vi "SDCP Receiver and Transmitter - Tx Table Updater.vi"(5 "Current Cell Position":T2, 7 "Entry position descriptors":cluster{"Start Row":i32, "End Row":i32}[](array[cluster]), 8 "error in (no error)":errorcluster, 10 "Table Control":refnum<vi>, 11 "Tx Table entry cluster array in":T1[](array[typedef])) -> (0 "error out":errorcluster, 3 "Tx Table entry cluster array out":T1[](array[typedef]))   [LabVIEW 2020]
uses:
  <vilib>/Utility/miscctls.llb/LVRowAndColumnTypeDef.ctl
  Typedefs/SDCP SMF Receiver and Transmitter - Transmit Table Element.ctl
  Typedefs/SDCP - Standard Message Frame Parameters - FGV - commands.ctl
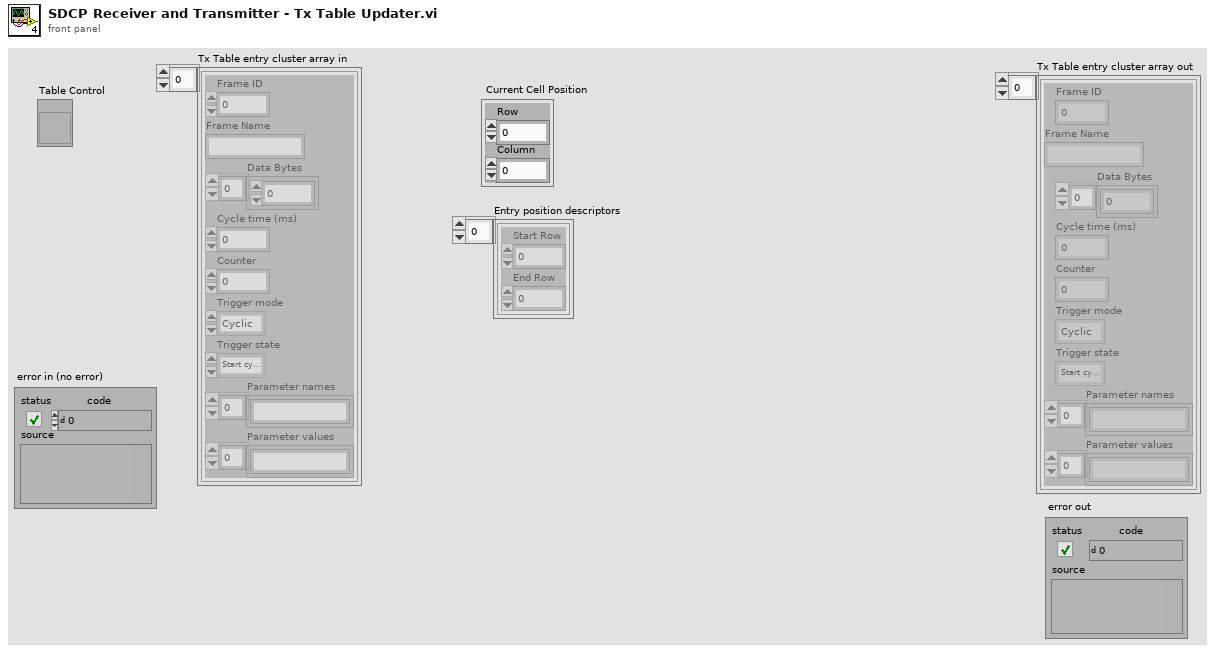
[diagram p1: front panel]
types:
  T1 = typedef "SDCP SMF Receiver and Transmitter - Transmit Table Element.ctl" = cluster{"Frame ID":i32, "Frame Name":string, "Data Bytes":u8[], "Cycle time (ms)":i32, "Counter":i32, "Trigger mode":enum16{"Triggered", "Cyclic"}, "Trigger state":enum16{"Stop cyclic trigger", "Start cyclic trigger", "Stop single trigger", "Start single trigger"}, "Parameter names":string[], "Parameter values":string[]}
  T2 = typedef "LVRowAndColumnTypeDef.ctl" = cluster{"Row":i32, "Column":i32}
  T3 = typedef "SDCP - Standard Message Frame Parameters - FGV - commands.ctl" = enum16{"Write descriptors", "Read descriptors", "Read values", "Load parameters from file", "Write values", "Read all descriptors"}
  T4 = enum16{"Stop cyclic trigger", "Start cyclic trigger", "Stop single trigger", "Start single trigger"}
  T5 = typedef "SDCP - SMF parameter descriptors.ctl" = cluster{"Frame name":string, "Frame ID":i32, "Data type":string, "Start Position":i32, "Length":i32, "Factor":dbl, "Offset":dbl, "Parameter name":string, "Value":string}
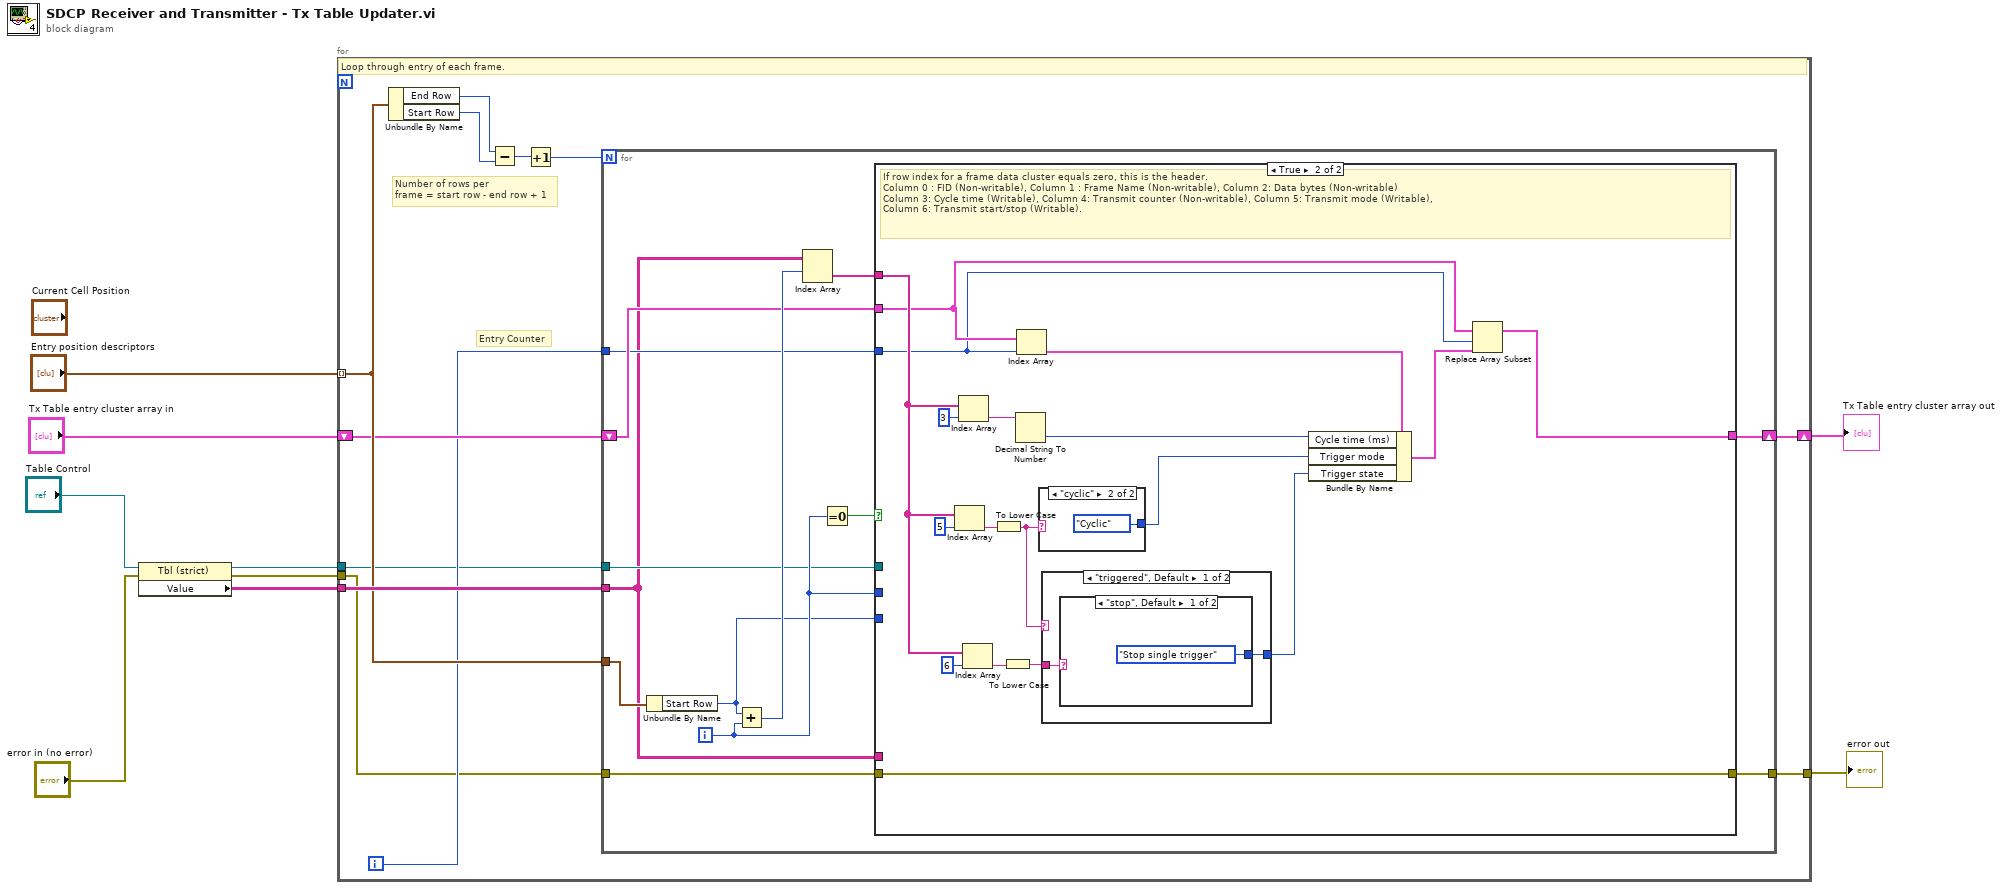
[diagram p0: block diagram]
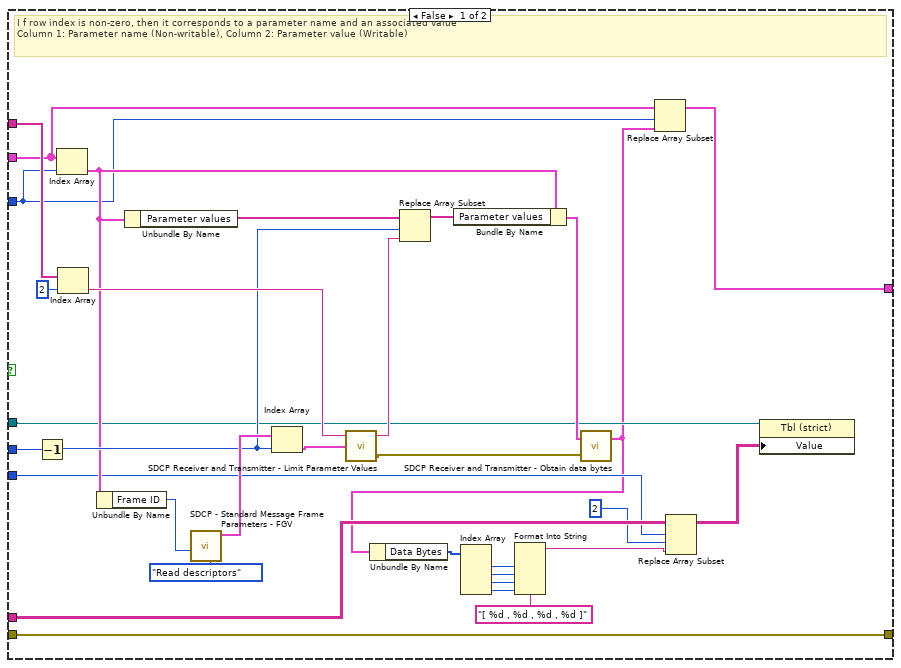
[diagram p2: hidden frame]
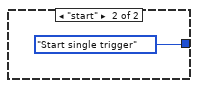
[diagram p3: hidden frame]
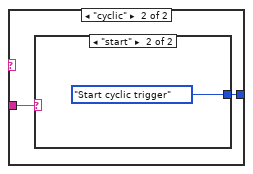
[diagram p4: hidden frame]
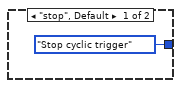
[diagram p5: hidden frame]
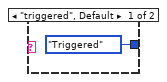
[diagram p6: hidden frame]
diagram:
  n1 = property class="Tbl (strict)"(reference="Table Control", error in="error in (no error)") -> (reference out=w1:refnum<vi>, error out=w7:errorcluster, "Value"=w6:string[][])
  n2 = for {
    tunnel: w6 -> [w17]
    tunnel: w7 -> [w12]
    tunnel: "Entry position descriptors" -> [w16] mode=indexing
    shift-right: [w13] -> w2
    shift-left: "Tx Table entry cluster array in" -> [w15]
    tunnel: [w11] -> w3
    tunnel: w1 -> [w10]
    i -> [w14]
    # "Entry Counter"
    # "Number of rows per\nframe = start row - end row + 1"
    # "Loop through entry of each frame."
    n3 = Unbundle By Name(w16) -> ("End Row"=w21:i32, "Start Row"=w20:i32)
    n4 = Subtract(x=w21, y=w20) -> (x-y=w19:i32)
    n5 = Increment(x=w19) -> (x+1=w18:i32)
    n6 = for {
      N: w18 -> [_]
      tunnel: w17 -> [w23]
      tunnel: w16 -> [w34]
      shift-right: [w28] -> w13
      shift-left: w15 -> [w30]
      tunnel: w14 -> [w29]
      tunnel: w12 -> [w26]
      tunnel: [w25] -> w11
      tunnel: w10 -> [w24]
      i -> [w27]
      n7 = Unbundle By Name(w34) -> ("Start Row"=w22:i32)
      n8 = Add(x=w22, y=w27) -> (x+y=w33:i32)
      n9 = Index Array(array=w23, index (row)=w33) -> (element=w31:string[])  [unwired: 1 in]
      n10 = Equal To 0?(x=w27) -> (x = 0?=w32:bool)
      n11 = case shown="True" w32 {
        tunnel: w31 -> [w62 w76]
        tunnel: w30 -> [w53 w73]
        tunnel: w29 -> [w52 w72]
        tunnel: [w51 w71] -> w28
        tunnel: w27 -> [w63 _]
        tunnel: w26 -> [w50 w70]
        tunnel: [w50 w70] -> w25
        tunnel: w24 -> [w46 _]
        tunnel: w23 -> [w47 _]
        tunnel: w22 -> [w44 _]
        frame False {
          # "I f row index is non-zero, then it corresponds to a parameter name and an associated value\nColumn 1: Parameter name (Non-writable), Column 2: Parameter value (Writable)"
          n12 = Decrement(x=w63) -> (x-1=w57:i32)
          n13 = Index Array(array=w53, index=w52) -> (element=w55:T1)
          n14 = Index Array(array=w62, index=2) -> (element=w59:string)
          n15 = Unbundle By Name(w55) -> ("Frame ID"=w65:i32)
          n16 = Unbundle By Name(w55) -> ("Parameter values"=w58:string[])
          n17 = call "SDCP - Standard Message Frame Parameters - FGV.vi"("FID"=w65, "Command"=SDCP_-_Standard_Message_Frame_Parameters_-_FGV_-_commands."Read descriptors") -> ("SMF Parameters descriptors out"=w64:T5[])  [unwired: 5 in, 1 out]
          n18 = Index Array(array=w64, index=w57) -> (element=w60:T5)
          n19 = call "SDCP Receiver and Transmitter - Limit Parameter Values.vi"("Parameter descriptor in"=w60, "Parameter value in"=w59) -> ("error out"=w49:errorcluster, "Parameter value out"=w56:string)  [unwired: 2 in]
          n20 = Replace Array Subset(array=w58, new element=w56, index=w57) -> (w54:string[])
          n21 = Bundle By Name(cluster=w55, "Parameter values"=w54) -> (w48:T1)
          n22 = call "SDCP Receiver and Transmitter - Obtain data bytes.vi"("error in (no error)"=w49, "Table element in"=w48) -> ("Table element out"=w42:T1)  [unwired: 1 out]
          n23 = Unbundle By Name(w42) -> ("Data Bytes"=w41:u8[])
          n24 = Index Array(array=w41) -> (element #1=w39:u8, element #2=w38:u8, element #3=w37:u8, element #4=w36:u8)  [unwired: 4 in]
          n25 = Format Into String(format string="[ %d , %d , %d , %d ]", w39, w38, w37, w36) -> (resulting string=w35:string)  [unwired: 2 in, 1 out]
          n26 = Replace Array Subset(array=w53, new element=w42, index=w52) -> (w51:T1[])
          n27 = Replace Array Subset(array=w47, new element=w35, index (row)=w44, index (col)=2 ("disabled index (col)")) -> (w45:string[][])
          n28 = property class="Tbl (strict)"(reference=w46, "Value"=w45) -> ()  [unwired: 1 in, 2 out]
        }
        frame True {
          # "If row index for a frame data cluster equals zero, this is the header. \nColumn 0 : FID (Non-writable), Column 1 : Frame Name (Non-writable), Column 2: Data bytes (Non-writable)\nColumn 3: Cycle time (Writable), Column 4: Transmit counter (Non-writable), Column 5: Transmit mode (Writable),\nColumn 6: Transmit start/stop (Writable)."
          n29 = Index Array(array=w76, index=5) -> (element=w80:string)
          n30 = Index Array(array=w76, index=3) -> (element=w83:string)
          n31 = Index Array(array=w76, index=6) -> (element=w75:string)
          n32 = To Lower Case(string=w80) -> (all lower case string=w78:string)
          n33 = To Lower Case(string=w75) -> (all lower case string=w74:string)
          n34 = Decimal String To Number(string=w83) -> (number=w82:i32)  [unwired: 2 in, 1 out]
          n35 = Index Array(array=w73, index=w72) -> (element=w69:T1)
          n36 = case shown="\"cyclic\"" w78 {
            tunnel: [enum16{"Triggered", "Cyclic"}."Triggered" ("Trigger mode") enum16{"Triggered", "Cyclic"}."Cyclic" ("Trigger mode")] -> w79
            frame "triggered", Default {
            }
            frame "cyclic" {
            }
          }
          n37 = case shown="\"triggered\", Default" w78 {
            tunnel: w74 -> [w86 w90]
            tunnel: [w85 w89] -> w67
            frame "triggered", Default {
              n38 = case shown="\"stop\", Default" w86 {
                tunnel: [T4."Stop single trigger" ("Trigger state") T4."Start single trigger" ("Trigger state")] -> w85
                frame "stop", Default {
                }
                frame "start" {
                }
              }
            }
            frame "cyclic" {
              n39 = case shown="\"start\"" w90 {
                tunnel: [T4."Stop cyclic trigger" ("Trigger state") T4."Start cyclic trigger" ("Trigger state")] -> w89
                frame "stop", Default {
                }
                frame "start" {
                }
              }
            }
          }
          n40 = Bundle By Name(cluster=w69, "Cycle time (ms)"=w82, "Trigger mode"=w79, "Trigger state"=w67) -> (w68:T1)
          n41 = Replace Array Subset(array=w73, new element=w68, index=w72) -> (w71:T1[])
        }
      }
    }
  }
  "Tx Table entry cluster array out" <- w2
  "error out" <- w3
